vi "Open HTML Report in Browser (Path).vi"(0 "path":path, 11 "error in (no error)":errorcluster) -> (4 "path out":path, 15 "error out":errorcluster)   [LabVIEW 2020, in "NI_ReportGenerationCore.lvlib"]
doc: "Displays an HTML report in the default Web browser. Wire data to the <B>report in</B> input to determine the polymorphic instance to use or manually select the instance."
uses:
  <vilib>/Utility/NIReport.llb/NI_ReportGenerationCore.lvlib
  <vilib>/Platform/browser.llb/Open URL in Default Browser (string).vi
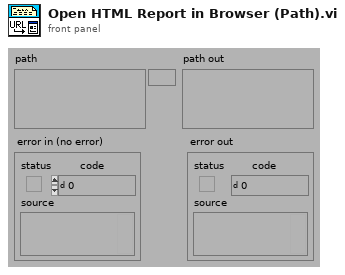
[diagram p1: front panel]
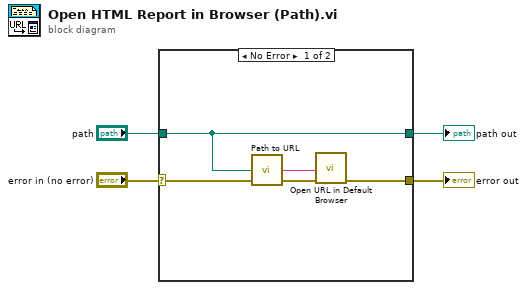
[diagram p0: block diagram]
diagram:
  n1 = case shown="No Error" "error in (no error)" {
    selector: "error in (no error)" -> [w6 w10]
    tunnel: [w7 w10] -> w3
    tunnel: "path" -> [w5 w9]
    tunnel: [w5 w9] -> w1
    frame No Error {
      n2 = call <vilib>:"Path to URL.vi"("path"=w5) -> ("url"=w8:string)
      n3 = call-poly <vilib>:"Open URL in Default Browser.vi"("error in (no error)"=w6, "URL"=w8) -> ("error out"=w7:errorcluster)  [unwired: 4 in, 1 out]
    }
    frame Error {
    }
  }
  "error out" <- w3
  "path out" <- w1
